vi "SetParameters.vi"(0 "Camera Reference in":refnum<k24>, 1 "error in (no error)":errorcluster, 3 "2D Exposure Mode (Timed Auto HDR Flash)":enum16{"Timed", "Auto", "HDR", "Flash"}(ring), 4 "2D Exposure Time (0.1-999)":dbl=0.1 min=0.1 max=999.0 step=0.1, 5 "2D Gray Value":i32 min=0 max=255 step=1, 7 "2D Auto-Exposure ROI (x, y, width, height)":T3, 8 "2D Tone Mapping":bool, 9 "2D HDR Exposure Count":i32=1 min=1 max=5 step=1, 10 "Ultra M ProcessingParams":T1={"DepthSmooth (Off Weak Normal Strong)"=enum."Normal", "\tDepthHoleFilling (Off Weak Normal Strong)"=enum."Normal", "\tDepthSurfaceNoiseRemoval (Off Weak Normal Strong)"=enum."Normal", "\t\tPhaseClusterOutlierRemoval (L0..L10)"=enum."L5", "\tSpuriousPhaseRemoval (Off Weak Normal Strong)"=enum."Normal", "\tLargeGradNoiseRemoval (Off Weak Normal Strong)"=enum."Normal", "\t\tPointCloudEdgePreservation (Sharp Normal Smooth)"=enum."Normal", "Group Exposure Selector"=enum."Exposure1", "Group Scan3D Exposure Time"=8.0, "Group Scan3D Gain"=2.0, "Group DLP Power Level"=80} {"Group DLP Power Level" min=0 max=100; "Group Scan3D Gain" min=0.0 max=16.0; "Group Scan3D Exposure Time" min=0.1 max=99.0}, 12 "2D HDR Exposure Sequence":T2={"Exposure 1"=0.1, "Exposure 2"=0.1, "Exposure 3"=0.1, "Exposure 4"=0.1, "Exposure 5"=0.1} {"Exposure 5" min=0.1 max=999.0; "Exposure 4" min=0.1 max=999.0; "Exposure 3" min=0.1 max=999.0; "Exposure 2" min=0.1 max=999.0; "Exposure 1" min=0.1 max=999.0}, 13 "3D Exposure Multiplier":i8=1 min=1 max=3 step=1, 14 "3D Exposure Sequence (value 0.1-99)":T4={"Exposure 1"=0.1, "Exposure 2"=0.1, "Exposure 3"=0.1} {"Exposure 3" min=0.1 max=99.0; "Exposure 2" min=0.1 max=99.0; "Exposure 1" min=0.1 max=99.0}, 15 "3D Gain (0-16)":dbl, 16 "Depth Range (lower upper)":cluster{"lower":i32, "upper":i32}, 17 "ROI (x, y, width, height)":T3, 23 "PointCloudSurfaceSmoothing (Off Weak Normal Strong)":u8(ring) items=["Off", "Weak", "Normal", "Strong"], 24 "PointCloudNoiseRemoval (Off Weak Normal Strong)":u8(ring) items=["Off", "Weak", "Normal", "Strong"], 25 "PointCloudOutlierRemoval (Off Weak Normal Strong)":u8(ring) items=["Off", "Weak", "Normal", "Strong"], 27 "Stripe Contrast Thresold (0-100)":i32 min=0 max=100 step=1) -> (20 "Camera Reference out":refnum<k24>, 21 "error out":errorcluster)   [LabVIEW 2023]
uses:
  C:/Program Files/National Instruments/LabVIEW 2025/MechEyeApiNet.dll
  Program Files/National Instruments/LabVIEW 2025/MechEyeApiNet.dll
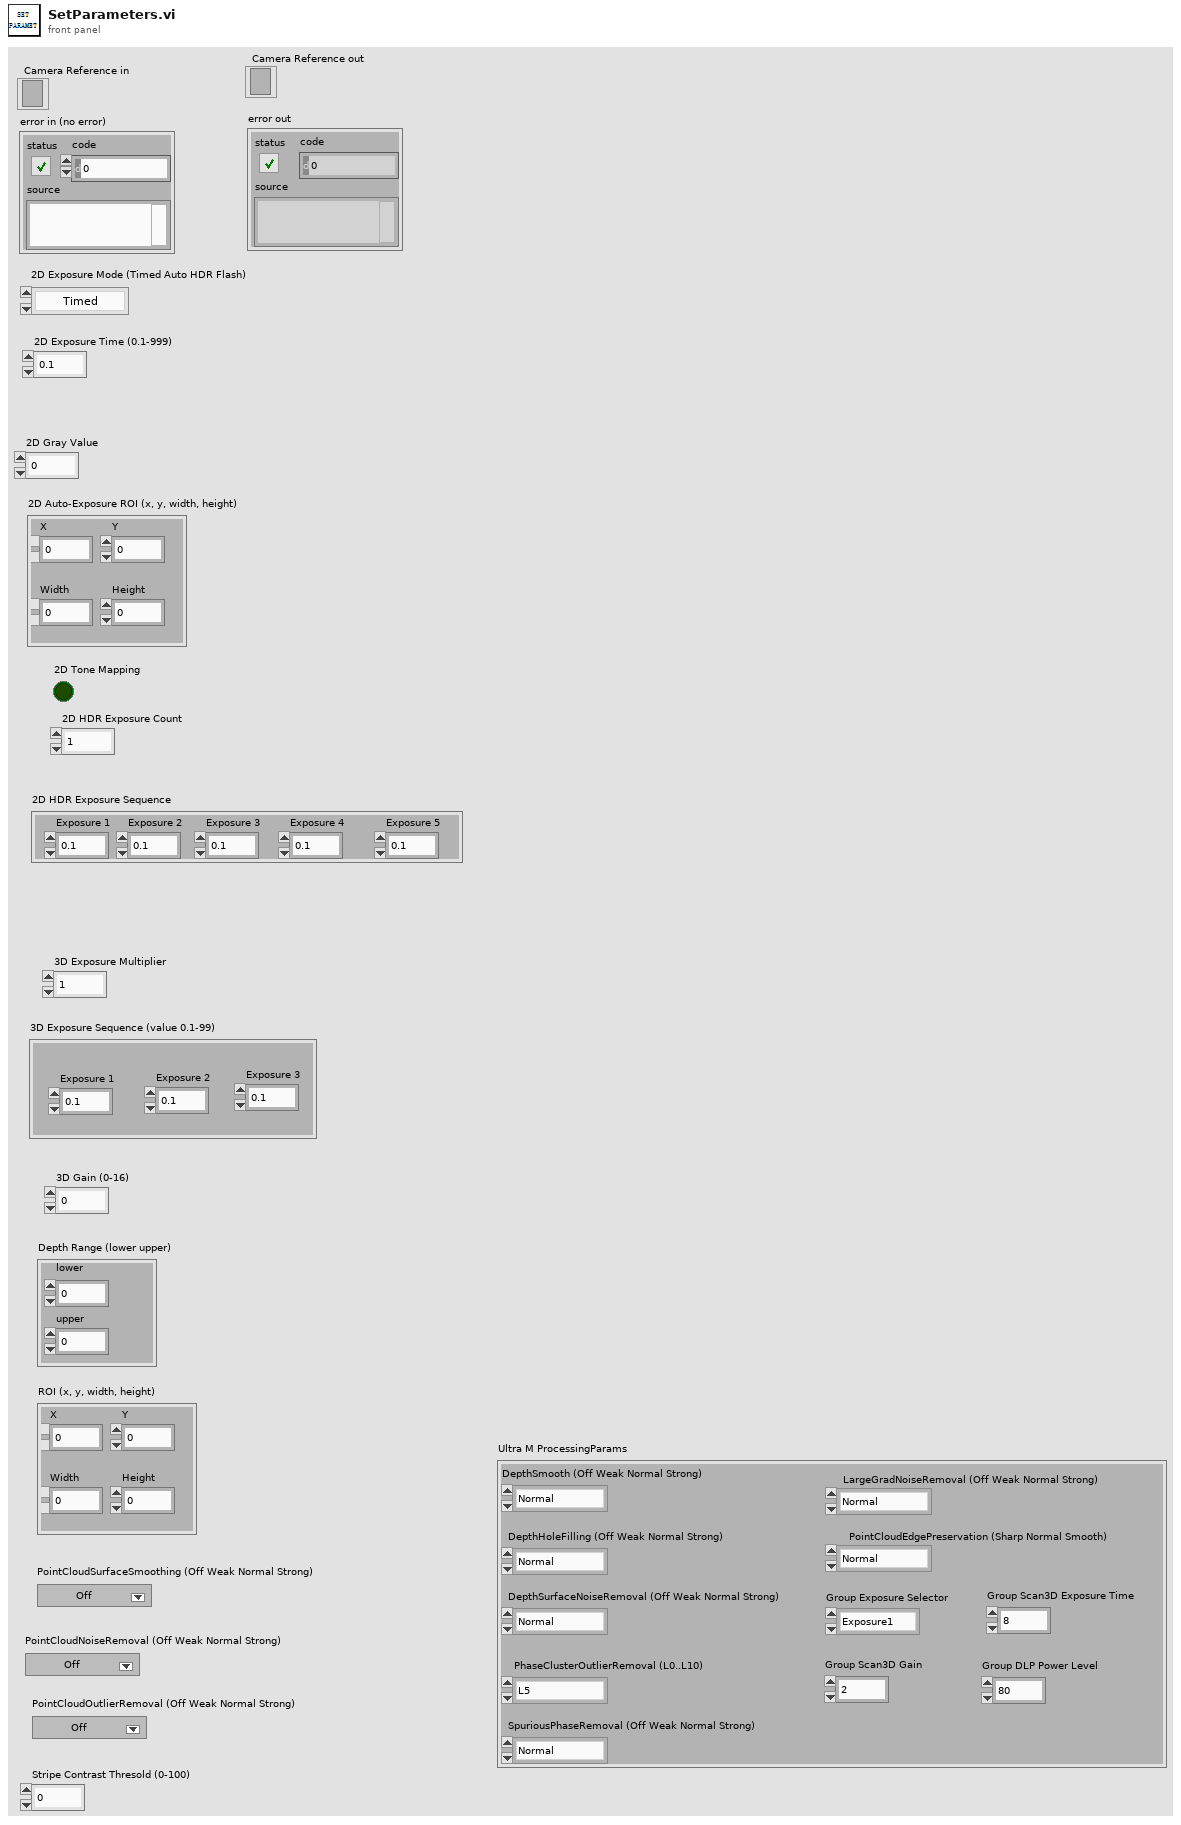
[diagram p1: front panel]
types:
  T1 = cluster{"DepthSmooth (Off Weak Normal Strong)":enum16{"Off", "Weak", "Normal", "Strong", ""}, "\tDepthHoleFilling (Off Weak Normal Strong)":enum16{"Off", "Weak", "Normal", "Strong", ""}, "\tDepthSurfaceNoiseRemoval (Off Weak Normal Strong)":enum16{"Off", "Weak", "Normal", "Strong", ""}, "\t\tPhaseClusterOutlierRemoval (L0..L10)":enum16{"L0", "L1", "L2", "L3", "L4", "L5", "L6", "L7", "L8", "L9", "L10"}, "\tSpuriousPhaseRemoval (Off Weak Normal Strong)":enum16{"Off", "Weak", "Normal", "Strong", ""}, "\tLargeGradNoiseRemoval (Off Weak Normal Strong)":enum16{"Off", "Weak", "Normal", "Strong", ""}, "\t\tPointCloudEdgePreservation (Sharp Normal Smooth)":enum16{"Sharp", "Normal", "Smooth"}, "Group Exposure Selector":enum16{"Exposure1", "Exposure2"}, "Group Scan3D Exposure Time":dbl, "Group Scan3D Gain":dbl, "Group DLP Power Level":i32}
  T2 = cluster{"Exposure 1":dbl, "Exposure 2":dbl, "Exposure 3":dbl, "Exposure 4":dbl, "Exposure 5":dbl}
  T3 = cluster{"X":i32, "Y":i32, "Width":i32, "Height":i32}
  T4 = cluster{"Exposure 1":dbl, "Exposure 2":dbl, "Exposure 3":dbl}
  T5 = enum16{"L0", "L1", "L2", "L3", "L4", "L5", "L6", "L7", "L8", "L9", "L10"}
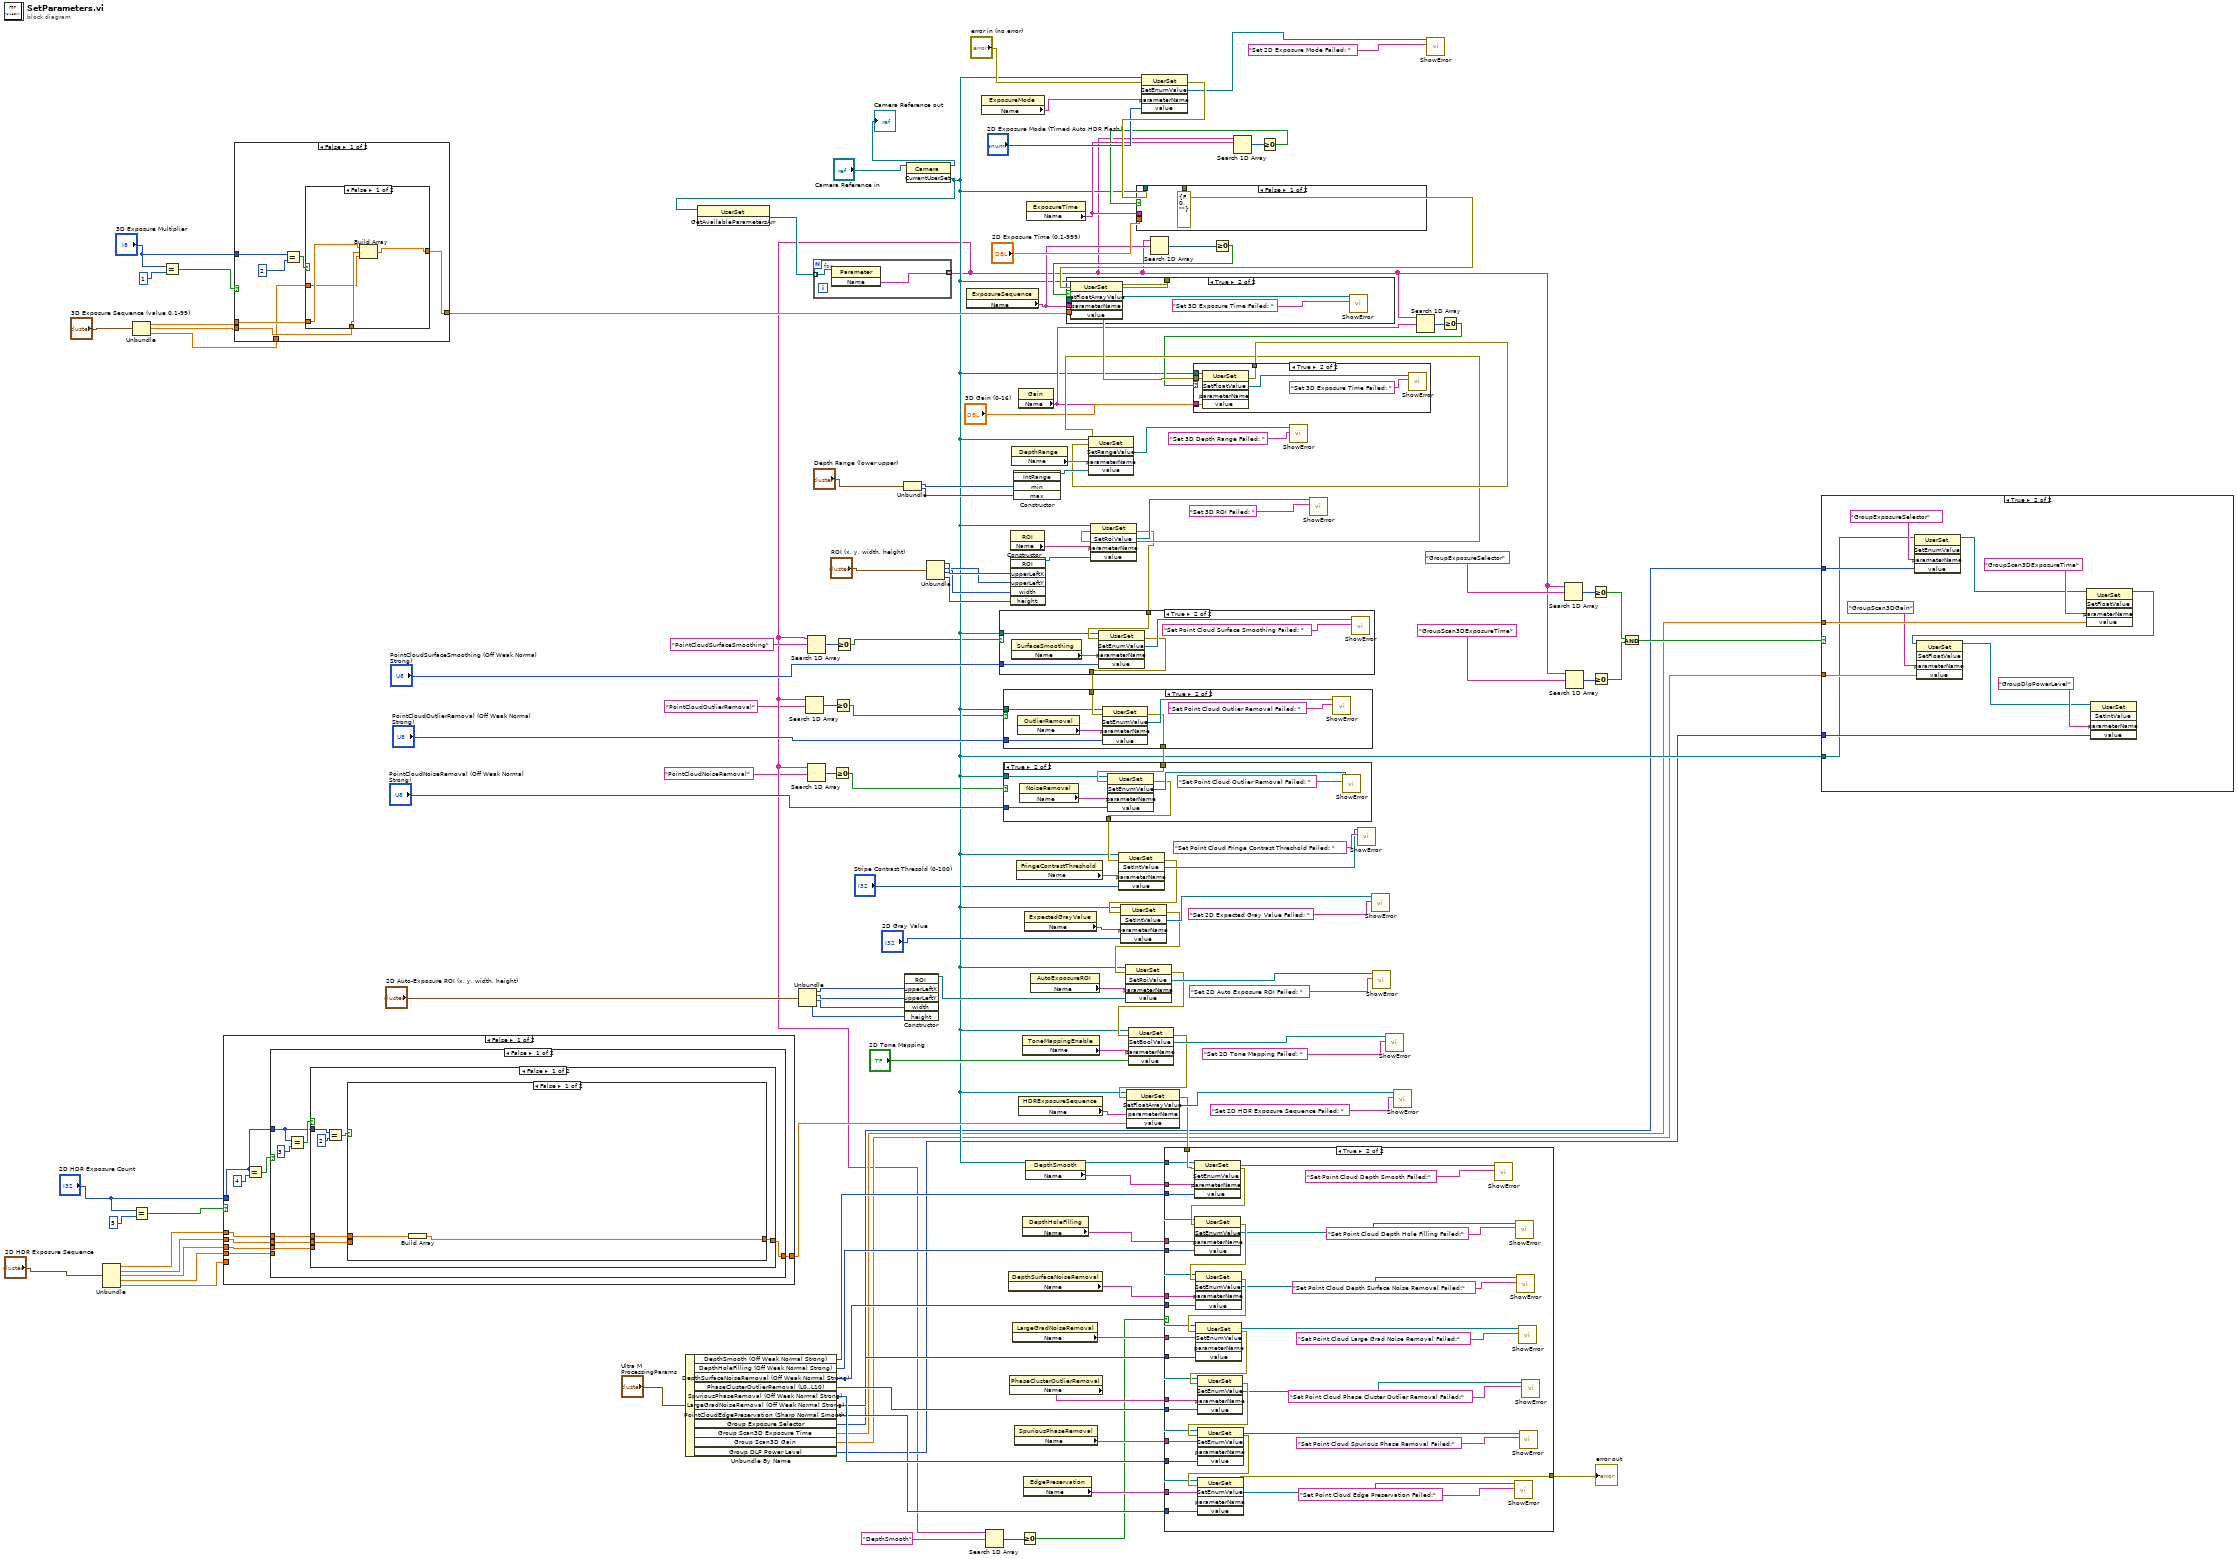
[diagram p0: block diagram]
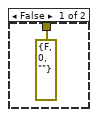
[diagram p7: hidden frame]
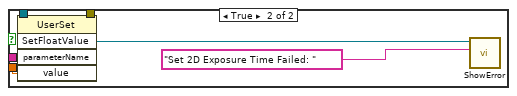
[diagram p8: hidden frame]
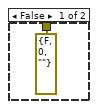
[diagram p9: hidden frame]
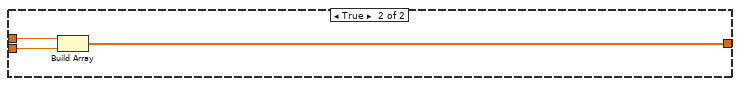
[diagram p10: hidden frame]
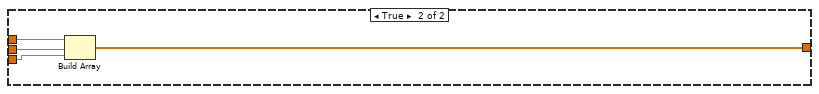
[diagram p11: hidden frame]
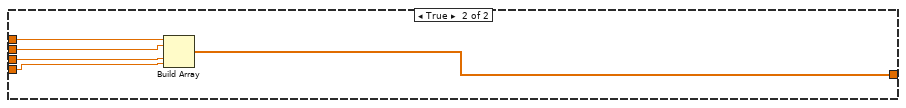
[diagram p12: hidden frame]
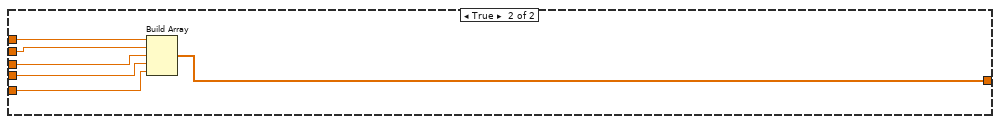
[diagram p13: hidden frame]
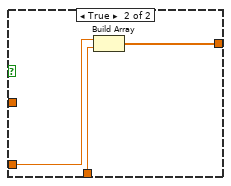
[diagram p14: hidden frame]
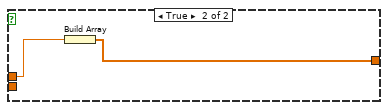
[diagram p15: hidden frame]
diagram:
  n1 = Unbundle("2D HDR Exposure Sequence") -> ("Exposure 1"=w65:dbl, "Exposure 2"=w64:dbl, "Exposure 3"=w63:dbl, "Exposure 4"=w58:dbl, "Exposure 5"=w57:dbl)
  n2 = Unbundle("3D Exposure Sequence (value 0.1-99)") -> ("Exposure 1"=w95:dbl, "Exposure 2"=w94:dbl, "Exposure 3"=w93:dbl)
  n3 = Equal?(x="2D HDR Exposure Count", y=5) -> (x = y?=w61:bool)
  n4 = Equal?(x="3D Exposure Multiplier", y=1) -> (x = y?=w90:bool)
  n5 = case shown="False" w61 {
    tunnel: w65 -> [w141 w176]
    tunnel: w64 -> [w140 w174]
    tunnel: w63 -> [w139 w173]
    tunnel: [w137 w175] -> w56
    tunnel: "2D HDR Exposure Count" -> [w136 _]
    tunnel: w58 -> [w138 w172]
    tunnel: w57 -> [_ w171]
    frame False {
      n6 = Equal?(x=w136, y=4) -> (x = y?=w142:bool)
      n7 = case shown="False" w142 {
        tunnel: w141 -> [w148 w170]
        tunnel: w140 -> [w147 w169]
        tunnel: w139 -> [w146 w168]
        tunnel: w138 -> [_ w167]
        tunnel: [w145 w166] -> w137
        tunnel: w136 -> [w144 _]
        frame False {
          n8 = Equal?(x=w144, y=3) -> (x = y?=w149:bool)
          n9 = case shown="False" w149 {
            tunnel: w148 -> [w153 w165]
            tunnel: w147 -> [w152 w164]
            tunnel: w146 -> [_ w163]
            tunnel: [w151 w162] -> w145
            tunnel: w144 -> [w156 _]
            frame False {
              n10 = Equal?(x=w156, y=2) -> (x = y?=w154:bool)
              n11 = case shown="False" w154 {
                tunnel: w153 -> [w158 w161]
                tunnel: w152 -> [_ w160]
                tunnel: [w157 w159] -> w151
                frame False {
                  n12 = Build Array(w158) -> (w157:dbl[])
                }
                frame True {
                  n13 = Build Array(w161, w160) -> (w159:dbl[])
                }
              }
            }
            frame True {
              n14 = Build Array(w165, w164, w163) -> (w162:dbl[])
            }
          }
        }
        frame True {
          n15 = Build Array(w170, w169, w168, w167) -> (w166:dbl[])
        }
      }
    }
    frame True {
      n16 = Build Array(w176, w174, w173, w172, w171) -> (w175:dbl[])
    }
  }
  n17 = case shown="False" w90 {
    tunnel: w95 -> [w180 w192]
    tunnel: w94 -> [w179 _]
    tunnel: w93 -> [w177 _]
    tunnel: [w178 w191] -> w92
    tunnel: "3D Exposure Multiplier" -> [w183 _]
    frame False {
      n18 = Equal?(x=w183, y=2) -> (x = y?=w181:bool)
      n19 = case shown="False" w181 {
        tunnel: w180 -> [w187 w190]
        tunnel: w179 -> [w186 w189]
        tunnel: [w184 w188] -> w178
        tunnel: w177 -> [w185 _]
        frame False {
          n20 = Build Array(w187, w186, w185) -> (w184:dbl[])
        }
        frame True {
          n21 = Build Array(w190, w189) -> (w188:dbl[])
        }
      }
    }
    frame True {
      n22 = Build Array(w192) -> (w191:dbl[])
    }
  }
  n23 = Unbundle By Name("Ultra M ProcessingParams") -> ("DepthSmooth (Off Weak Normal Strong)"=w24:enum16{"Off", "Weak", "Normal", "Strong", ""}, "DepthHoleFilling (Off Weak Normal Strong)"=w23:enum16{"Off", "Weak", "Normal", "Strong", ""}, "DepthSurfaceNoiseRemoval (Off Weak Normal Strong)"=w22:enum16{"Off", "Weak", "Normal", "Strong", ""}, "PhaseClusterOutlierRemoval (L0..L10)"=w21:T5, "SpuriousPhaseRemoval (Off Weak Normal Strong)"=w20:enum16{"Off", "Weak", "Normal", "Strong", ""}, "LargeGradNoiseRemoval (Off Weak Normal Strong)"=w19:enum16{"Off", "Weak", "Normal", "Strong", ""}, "PointCloudEdgePreservation (Sharp Normal Smooth)"=w18:enum16{"Sharp", "Normal", "Smooth"}, "Group Exposure Selector"=w14:enum16{"Exposure1", "Exposure2"}, "Group Scan3D Exposure Time"=w13:dbl, "Group Scan3D Gain"=w12:dbl, "Group DLP Power Level"=w11:i32)
  n24 = Unbundle("2D Auto-Exposure ROI (x, y, width, height)") -> ("X"=w82:i32, "Y"=w81:i32, "Width"=w80:i32, "Height"=w79:i32)
  n25 = Unbundle("Depth Range (lower upper)") -> ("lower"=w101:i32, "upper"=w100:i32)
  n26 = constructor class="ROI"("upperLeftX"=w82, "upperLeftY"=w81, "width"=w80, "height"=w79) -> (reference out=w78:refnum<k24>)  [unwired: 3 in, 6 out]
  n27 = invoke class="Camera" method="CurrentUserSet"(reference="Camera Reference in") -> (reference out=→"Camera Reference out":refnum<k24>, "CurrentUserSet"=w30:refnum<k24>)  [unwired: 2 in, 1 out]
  n28 = invoke class="UserSet" method="GetAvailableParametersArr"(reference=w30) -> ("GetAvailableParametersArr"=w53:refnum<k24>[])  [unwired: 2 in, 2 out]
  n29 = for {
    tunnel: w53 -> [w194] mode=indexing
    tunnel: [w193] -> w9 mode=indexing
    n30 = invoke class="Parameter" method="Name"(reference=w194) -> ("Name"=w193:string)  [unwired: 2 in, 2 out]
  }
  n31 = Search 1D Array(1D array=w9, element="PointCloudOutlierRemoval") -> (index of element=w5:i32)  [unwired: 1 in]
  n32 = Search 1D Array(1D array=w9, element="PointCloudSurfaceSmoothing") -> (index of element=w6:i32)  [unwired: 1 in]
  n33 = Search 1D Array(1D array=w9, element="PointCloudNoiseRemoval") -> (index of element=w4:i32)  [unwired: 1 in]
  n34 = Greater Or Equal To 0?(x=w4) -> (x >= 0?=w1:bool)
  n35 = Greater Or Equal To 0?(x=w5) -> (x >= 0?=w2:bool)
  n36 = Greater Or Equal To 0?(x=w6) -> (x >= 0?=w3:bool)
  n37 = Unbundle("ROI (x, y, width, height)") -> ("X"=w106:i32, "Y"=w105:i32, "Width"=w104:i32, "Height"=w103:i32)
  n38 = property class="ExposureSequence"() -> ("Name"=w52:string)  [unwired: 2 in, 2 out]
  n39 = property class="ExposureMode"() -> ("Name"=w130:string)  [unwired: 2 in, 2 out]
  n40 = Search 1D Array(1D array=w9, element="DepthSmooth") -> (index of element=w16:i32)  [unwired: 1 in]
  n41 = property class="DepthSurfaceNoiseRemoval"() -> ("Name"=w32:string)  [unwired: 2 in, 2 out]
  n42 = property class="PhaseClusterOutlierRemoval"() -> ("Name"=w29:string)  [unwired: 2 in, 2 out]
  n43 = property class="ROI"() -> ("Name"=w122:string)  [unwired: 2 in, 2 out]
  n44 = constructor class="ROI"("upperLeftX"=w106, "upperLeftY"=w105, "width"=w104, "height"=w103) -> (reference out=w121:refnum<k24>)  [unwired: 3 in, 6 out]
  n45 = property class="DepthRange"() -> ("Name"=w129:string)  [unwired: 2 in, 2 out]
  n46 = property class="LargeGradNoiseRemoval"() -> ("Name"=w31:string)  [unwired: 2 in, 2 out]
  n47 = constructor class="IntRange"("min"=w101, "max"=w100) -> (reference out=w128:refnum<k24>)  [unwired: 3 in, 4 out]
  n48 = property class="SpuriousPhaseRemoval"() -> ("Name"=w28:string)  [unwired: 2 in, 2 out]
  n49 = property class="FringeContrastThreshold"() -> ("Name"=w111:string)  [unwired: 2 in, 2 out]
  n50 = property class="Gain"() -> ("Name"=w45:string)  [unwired: 2 in, 2 out]
  n51 = property class="HDRExposureSequence"() -> ("Name"=w66:string)  [unwired: 2 in, 2 out]
  n52 = Greater Or Equal To 0?(x=w16) -> (x >= 0?=w15:bool)
  n53 = property class="ToneMappingEnable"() -> ("Name"=w74:string)  [unwired: 2 in, 2 out]
  n54 = property class="DepthHoleFilling"() -> ("Name"=w33:string)  [unwired: 2 in, 2 out]
  n55 = property class="EdgePreservation"() -> ("Name"=w27:string)  [unwired: 2 in, 2 out]
  n56 = property class="ExpectedGrayValue"() -> ("Name"=w87:string)  [unwired: 2 in, 2 out]
  n57 = property class="DepthSmooth"() -> ("Name"=w36:string)  [unwired: 2 in, 2 out]
  n58 = property class="ExposureTime"() -> ("Name"=w48:string)  [unwired: 2 in, 2 out]
  n59 = property class="AutoExposureROI"() -> ("Name"=w75:string)  [unwired: 2 in, 2 out]
  n60 = invoke class="UserSet" method="SetEnumValue"(reference=w30, error in="error in (no error)", "parameterName"=w130, "value"="2D Exposure Mode (Timed Auto HDR Flash)") -> (error out=w134:errorcluster, "SetEnumValue"=w132:refnum<k24>)  [unwired: 1 in, 3 out]
  n61 = Search 1D Array(1D array=w9, element=w52) -> (index of element=w51:i32)  [unwired: 1 in]
  n62 = Greater Or Equal To 0?(x=w51) -> (x >= 0?=w50:bool)
  n63 = Search 1D Array(1D array=w9, element=w48) -> (index of element=w49:i32)  [unwired: 1 in]
  n64 = Greater Or Equal To 0?(x=w49) -> (x >= 0?=w47:bool)
  n65 = case shown="False" w47 {
    tunnel: w134 -> [_ w202]
    tunnel: [errorcluster {"status"=FALSE, "code"=0, "source"=""} ("error out") w199] -> w125
    tunnel: "2D Exposure Time (0.1-999)" -> [_ w198]
    tunnel: w30 -> [_ w197]
    tunnel: w48 -> [_ w196]
    frame False {
    }
    frame True {
      n66 = invoke class="UserSet" method="SetFloatValue"(reference=w197, error in=w202, "parameterName"=w196, "value"=w198) -> (error out=w199:errorcluster, "SetFloatValue"=w200:refnum<k24>)  [unwired: 1 in, 3 out]
      n67 = call "ShowError.vi"("String"="Set 2D Exposure Time Failed: ", "MMind.Eye.ErrorStatus"=w200) -> ()  [unwired: 10 in]
    }
  }
  n68 = case shown="True" w50 {
    tunnel: w125 -> [_ w208]
    tunnel: [errorcluster {"status"=FALSE, "code"=0, "source"=""} ("error out") w207] -> w124
    tunnel: w92 -> [_ w206]
    tunnel: w30 -> [_ w205]
    tunnel: w52 -> [_ w204]
    frame False {
    }
    frame True {
      n69 = invoke class="UserSet" method="SetFloatArrayValue"(reference=w205, error in=w208, "parameterName"=w204, "value"=w206) -> (error out=w207:errorcluster, "SetFloatArrayValue"=w209:refnum<k24>)  [unwired: 1 in, 3 out]
      n70 = call "ShowError.vi"("String"="Set 3D Exposure Time Failed: ", "MMind.Eye.ErrorStatus"=w209) -> ()  [unwired: 10 in]
    }
  }
  n71 = Search 1D Array(1D array=w9, element=w45) -> (index of element=w46:i32)  [unwired: 1 in]
  n72 = call "ShowError.vi"("String"="Set 2D Exposure Mode Failed: ", "MMind.Eye.ErrorStatus"=w132) -> ()  [unwired: 10 in]
  n73 = Greater Or Equal To 0?(x=w46) -> (x >= 0?=w44:bool)
  n74 = case shown="True" w44 {
    tunnel: w124 -> [_ w216]
    tunnel: [errorcluster {"status"=FALSE, "code"=0, "source"=""} ("error out") w215] -> w123
    tunnel: "3D Gain (0-16)" -> [_ w214]
    tunnel: w30 -> [_ w213]
    tunnel: w45 -> [_ w212]
    frame False {
    }
    frame True {
      n75 = invoke class="UserSet" method="SetFloatValue"(reference=w213, error in=w216, "parameterName"=w212, "value"=w214) -> (error out=w215:errorcluster, "SetFloatValue"=w217:refnum<k24>)  [unwired: 1 in, 3 out]
      n76 = call "ShowError.vi"("String"="Set 3D Exposure Time Failed: ", "MMind.Eye.ErrorStatus"=w217) -> ()  [unwired: 10 in]
    }
  }
  n77 = invoke class="UserSet" method="SetRangeValue"(reference=w30, error in=w123, "parameterName"=w129, "value"=w128) -> (error out=w120:errorcluster, "SetRangeValue"=w126:refnum<k24>)  [unwired: 1 in, 3 out]
  n78 = invoke class="UserSet" method="SetRoiValue"(reference=w30, error in=w120, "parameterName"=w122, "value"=w121) -> (error out=w117:errorcluster, "SetRoiValue"=w118:refnum<k24>)  [unwired: 1 in, 3 out]
  n79 = case shown="True" w3 {
    tunnel: w117 -> [w219 w223]
    tunnel: [w219 w222] -> w116
    tunnel: "PointCloudSurfaceSmoothing (Off Weak Normal Strong)" -> [_ w221]
    tunnel: w30 -> [_ w220]
    frame False {
    }
    frame True {
      n80 = property class="SurfaceSmoothing"() -> ("Name"=w226:string)  [unwired: 2 in, 2 out]
      n81 = invoke class="UserSet" method="SetEnumValue"(reference=w220, error in=w223, "parameterName"=w226, "value"=w221) -> (error out=w222:errorcluster, "SetEnumValue"=w224:refnum<k24>)  [unwired: 1 in, 3 out]
      n82 = call "ShowError.vi"("String"="Set Point Cloud Surface Smoothing Failed: ", "MMind.Eye.ErrorStatus"=w224) -> ()  [unwired: 10 in]
    }
  }
  n83 = case shown="True" w2 {
    tunnel: w116 -> [w227 w231]
    tunnel: [w227 w230] -> w115
    tunnel: "PointCloudOutlierRemoval (Off Weak Normal Strong)" -> [_ w229]
    tunnel: w30 -> [_ w228]
    frame False {
    }
    frame True {
      n84 = property class="OutlierRemoval"() -> ("Name"=w234:string)  [unwired: 2 in, 2 out]
      n85 = invoke class="UserSet" method="SetEnumValue"(reference=w228, error in=w231, "parameterName"=w234, "value"=w229) -> (error out=w230:errorcluster, "SetEnumValue"=w232:refnum<k24>)  [unwired: 1 in, 3 out]
      n86 = call "ShowError.vi"("String"="Set Point Cloud Outlier Removal Failed: ", "MMind.Eye.ErrorStatus"=w232) -> ()  [unwired: 10 in]
    }
  }
  n87 = case shown="True" w1 {
    tunnel: w115 -> [w235 w239]
    tunnel: [w235 w238] -> w114
    tunnel: "PointCloudNoiseRemoval (Off Weak Normal Strong)" -> [_ w237]
    tunnel: w30 -> [_ w236]
    frame False {
    }
    frame True {
      n88 = property class="NoiseRemoval"() -> ("Name"=w242:string)  [unwired: 2 in, 2 out]
      n89 = invoke class="UserSet" method="SetEnumValue"(reference=w236, error in=w239, "parameterName"=w242, "value"=w237) -> (error out=w238:errorcluster, "SetEnumValue"=w240:refnum<k24>)  [unwired: 1 in, 3 out]
      n90 = call "ShowError.vi"("String"="Set Point Cloud Outlier Removal Failed: ", "MMind.Eye.ErrorStatus"=w240) -> ()  [unwired: 10 in]
    }
  }
  n91 = invoke class="UserSet" method="SetIntValue"(reference=w30, error in=w114, "parameterName"=w111, "value"="Stripe Contrast Thresold (0-100)") -> (error out=w70:errorcluster, "SetIntValue"=w112:refnum<k24>)  [unwired: 1 in, 3 out]
  n92 = invoke class="UserSet" method="SetIntValue"(reference=w30, error in=w70, "parameterName"=w87, "value"="2D Gray Value") -> (error out=w69:errorcluster, "SetIntValue"=w84:refnum<k24>)  [unwired: 1 in, 3 out]
  n93 = invoke class="UserSet" method="SetRoiValue"(reference=w30, error in=w69, "parameterName"=w75, "value"=w78) -> (error out=w68:errorcluster, "SetRoiValue"=w76:refnum<k24>)  [unwired: 1 in, 3 out]
  n94 = invoke class="UserSet" method="SetBoolValue"(reference=w30, error in=w68, "parameterName"=w74, "value"="2D Tone Mapping") -> (error out=w67:errorcluster, "SetBoolValue"=w71:refnum<k24>)  [unwired: 1 in, 3 out]
  n95 = invoke class="UserSet" method="SetFloatArrayValue"(reference=w30, error in=w67, "parameterName"=w66, "value"=w56) -> (error out=w35:errorcluster, "SetFloatArrayValue"=w54:refnum<k24>)  [unwired: 1 in, 3 out]
  n96 = case shown="True" w15 {
    tunnel: w36 -> [_ w280]
    tunnel: w35 -> [w243 w279]
    tunnel: [w243 w272] -> w34
    tunnel: w33 -> [_ w271]
    tunnel: w32 -> [_ w270]
    tunnel: w31 -> [_ w269]
    tunnel: w30 -> [_ w268]
    tunnel: w29 -> [_ w267]
    tunnel: w28 -> [_ w266]
    tunnel: w27 -> [_ w265]
    tunnel: w24 -> [_ w264]
    tunnel: w23 -> [_ w263]
    tunnel: w22 -> [_ w262]
    tunnel: w21 -> [_ w261]
    tunnel: w20 -> [_ w260]
    tunnel: w19 -> [_ w259]
    tunnel: w18 -> [_ w258]
    frame False {
    }
    frame True {
      n97 = invoke class="UserSet" method="SetEnumValue"(reference=w268, error in=w279, "parameterName"=w280, "value"=w264) -> (error out=w278:errorcluster, "SetEnumValue"=w256:refnum<k24>)  [unwired: 1 in, 3 out]
      n98 = invoke class="UserSet" method="SetEnumValue"(reference=w268, error in=w278, "parameterName"=w271, "value"=w263) -> (error out=w277:errorcluster, "SetEnumValue"=w249:refnum<k24>)  [unwired: 1 in, 3 out]
      n99 = invoke class="UserSet" method="SetEnumValue"(reference=w268, error in=w277, "parameterName"=w270, "value"=w262) -> (error out=w276:errorcluster, "SetEnumValue"=w248:refnum<k24>)  [unwired: 1 in, 3 out]
      n100 = invoke class="UserSet" method="SetEnumValue"(reference=w268, error in=w276, "parameterName"=w269, "value"=w259) -> (error out=w275:errorcluster, "SetEnumValue"=w247:refnum<k24>)  [unwired: 1 in, 3 out]
      n101 = invoke class="UserSet" method="SetEnumValue"(reference=w268, error in=w275, "parameterName"=w267, "value"=w261) -> (error out=w274:errorcluster, "SetEnumValue"=w246:refnum<k24>)  [unwired: 1 in, 3 out]
      n102 = invoke class="UserSet" method="SetEnumValue"(reference=w268, error in=w274, "parameterName"=w266, "value"=w260) -> (error out=w273:errorcluster, "SetEnumValue"=w245:refnum<k24>)  [unwired: 1 in, 3 out]
      n103 = invoke class="UserSet" method="SetEnumValue"(reference=w268, error in=w273, "parameterName"=w265, "value"=w258) -> (error out=w272:errorcluster, "SetEnumValue"=w244:refnum<k24>)  [unwired: 1 in, 3 out]
      n104 = call "ShowError.vi"("String"="Set Point Cloud Depth Smooth Failed:", "MMind.Eye.ErrorStatus"=w256) -> ()  [unwired: 10 in]
      n105 = call "ShowError.vi"("String"="Set Point Cloud Edge Preservation Failed:", "MMind.Eye.ErrorStatus"=w244) -> ()  [unwired: 10 in]
      n106 = call "ShowError.vi"("String"="Set Point Cloud Depth Hole Filling Failed:", "MMind.Eye.ErrorStatus"=w249) -> ()  [unwired: 10 in]
      n107 = call "ShowError.vi"("String"="Set Point Cloud Depth Surface Noise Removal Failed:", "MMind.Eye.ErrorStatus"=w248) -> ()  [unwired: 10 in]
      n108 = call "ShowError.vi"("String"="Set Point Cloud Large Grad Noise Removal Failed:", "MMind.Eye.ErrorStatus"=w247) -> ()  [unwired: 10 in]
      n109 = call "ShowError.vi"("String"="Set Point Cloud Spurious Phase Removal Failed:", "MMind.Eye.ErrorStatus"=w245) -> ()  [unwired: 10 in]
      n110 = call "ShowError.vi"("String"="Set Point Cloud Phase Cluster Outlier Removal Failed:", "MMind.Eye.ErrorStatus"=w246) -> ()  [unwired: 10 in]
    }
  }
  "error out" <- w34
  n111 = call "ShowError.vi"("String"="Set 3D Depth Range Failed: ", "MMind.Eye.ErrorStatus"=w126) -> ()  [unwired: 10 in]
  n112 = call "ShowError.vi"("String"="Set 3D ROI Failed: ", "MMind.Eye.ErrorStatus"=w118) -> ()  [unwired: 10 in]
  n113 = call "ShowError.vi"("String"="Set Point Cloud Fringe Contrast Threshold Failed: ", "MMind.Eye.ErrorStatus"=w112) -> ()  [unwired: 10 in]
  n114 = call "ShowError.vi"("String"="Set 2D Expected Gray Value Failed: ", "MMind.Eye.ErrorStatus"=w84) -> ()  [unwired: 10 in]
  n115 = call "ShowError.vi"("String"="Set 2D Auto Exposure ROI Failed: ", "MMind.Eye.ErrorStatus"=w76) -> ()  [unwired: 10 in]
  n116 = call "ShowError.vi"("String"="Set 2D Tone Mapping Failed: ", "MMind.Eye.ErrorStatus"=w71) -> ()  [unwired: 10 in]
  n117 = call "ShowError.vi"("String"="Set 2D HDR Exposure Sequence Failed: ", "MMind.Eye.ErrorStatus"=w54) -> ()  [unwired: 10 in]
  n118 = Search 1D Array(1D array=w9, element="GroupExposureSelector") -> (index of element=w41:i32)  [unwired: 1 in]
  n119 = Search 1D Array(1D array=w9, element="GroupScan3DExposureTime") -> (index of element=w40:i32)  [unwired: 1 in]
  n120 = Greater Or Equal To 0?(x=w41) -> (x >= 0?=w39:bool)
  n121 = Greater Or Equal To 0?(x=w40) -> (x >= 0?=w38:bool)
  n122 = And(x=w39, y=w38) -> (x .and. y?=w37:bool)
  n123 = case shown="True" w37 {
    tunnel: w30 -> [_ w284]
    tunnel: w14 -> [_ w291]
    tunnel: w13 -> [_ w290]
    tunnel: w12 -> [_ w289]
    tunnel: w11 -> [_ w288]
    frame False {
    }
    frame True {
      n124 = invoke class="UserSet" method="SetEnumValue"(reference=w284, "parameterName"="GroupExposureSelector", "value"=w291) -> (reference out=w283:refnum<k24>)  [unwired: 2 in, 4 out]
      n125 = invoke class="UserSet" method="SetFloatValue"(reference=w283, "parameterName"="GroupScan3DExposureTime", "value"=w290) -> (reference out=w282:refnum<k24>)  [unwired: 2 in, 4 out]
      n126 = invoke class="UserSet" method="SetFloatValue"(reference=w282, "parameterName"="GroupScan3DGain", "value"=w289) -> (reference out=w281:refnum<k24>)  [unwired: 2 in, 4 out]
      n127 = invoke class="UserSet" method="SetIntValue"(reference=w281, "parameterName"="GroupDlpPowerLevel", "value"=w288) -> ()  [unwired: 2 in, 5 out]
    }
  }
